vi "lvlauncher.vi"   [LabVIEW 2013]
uses:
  constants/arguments.ctl
  kernel32.dll
types:
  T1 = typedef "arguments.ctl" = cluster{"working directory":string, "flags":string[], "values":string[]}
  T2 = enum32{"invalid app kind", "Development System", "Run Time System", "Student Edition", "Embedded LabVIEW", "Evaluation", "Custom"}
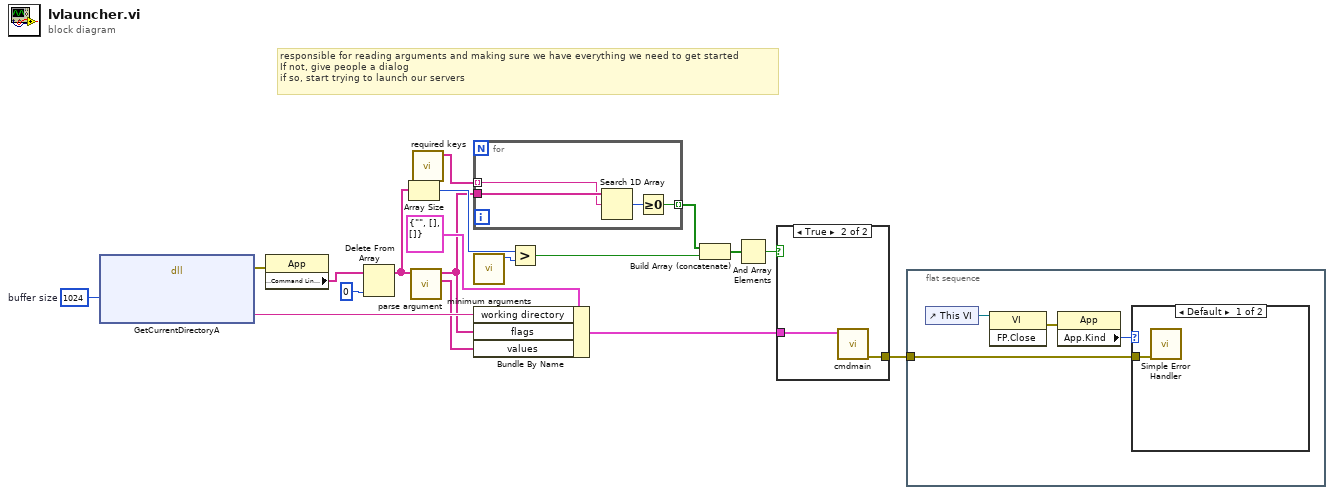
[diagram p0: block diagram]
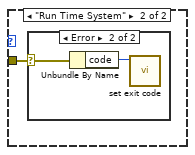
[diagram p2: hidden frame]
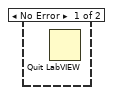
[diagram p3: hidden frame]
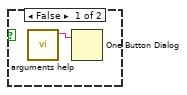
[diagram p4: hidden frame]
diagram:
  w17 = 1024  # buffer size
  # "responsible for reading arguments and making sure we have everything we need to get started\nIf not, give people a dialog\nif so, start trying to launch our servers"
  n1 = dll-call lib="kernel32.dll" fn="GetCurrentDirectoryA" ("Kernel32.dll - \nGetCurrentDirectoryA")("nBufferLength"=w17) -> (error out=w15:errorcluster, "lpBuffer"=w4:string)  [unwired: 5 in, 2 out]
  n2 = property class="App"(error in=w15) -> ("Application:Command Line Arguments"=w18:string[])  [unwired: 1 in, 2 out]
  n3 = Delete From Array(array=w18, index=0) -> (array with subset deleted=w11:string[])  [unwired: 1 in, 1 out]
  n4 = Array Size(array=w11) -> (size(s)=w12:i32)
  n5 = call "parse argument.vi"("Arguments"=w11) -> ("values"=w1:string[], "flags"=w2:string[])  [unwired: 9 in]
  n6 = call "required keys.vi"() -> ("required keys"=w10:string[])  [unwired: 11 in]
  n7 = for {
    tunnel: w2 -> [w22]
    tunnel: w10 -> [w21] mode=indexing
    tunnel: [w19] -> w9 mode=indexing
    n8 = Search 1D Array(1D array=w22, element=w21) -> (index of element=w20:i32)  [unwired: 1 in]
    n9 = Greater Or Equal To 0?(x=w20) -> (x >= 0?=w19:bool)
  }
  n10 = call "minimum arguments.vi"() -> ("minimum arguments"=w13:i32)  [unwired: 11 in]
  n11 = Bundle By Name(cluster=T1 {"working directory"="", "flags"=[], "values"=[]} ("command line arguments"), "working directory"=w4, "flags"=w2, "values"=w1) -> (w3:T1)
  n12 = Greater?(x=w12, y=w13) -> (0:w7:bool)
  n13 = Build Array (concatenate)(w9, w7) -> (w8:bool[])
  n14 = And Array Elements(Boolean array=w8) -> (logical AND=w6:bool)
  n15 = case shown="True" w6 {
    tunnel: [_ w25] -> w14
    tunnel: w3 -> [_ w24]
    frame False {
      n16 = call "arguments help.vi"() -> ("args help"=w23:string)  [unwired: 11 in]
      n17 = One Button Dialog(message=w23) -> ()  [unwired: 1 in, 1 out]
    }
    frame True {
      n18 = call "cmdmain.vi"("command line arguments"=w24) -> ("error out"=w25:errorcluster)  [unwired: 10 in]
    }
  }
  n19 = flat-sequence {
    tunnel: w14 -> [w26]
    frame #0 {
      n20 = control-ref of="This VI"() -> (w27:refnum<vi>)
      n21 = invoke class="VI" method="FP.Close"(reference=w27) -> (error out=w28:errorcluster)  [unwired: 2 in, 2 out]
      n22 = property class="App"(error in=w28) -> ("App.Kind"=w29:T2)  [unwired: 1 in, 2 out]
      n23 = case shown="Default" w29 {
        tunnel: w26 -> [w30 w31]
        frame Default {
          n24 = call <vilib>:"Simple Error Handler.vi"("error in (no error)"=w30) -> ()  [unwired: 4 in, 5 out]
        }
        frame "Run Time System" {
          n25 = case shown="Error" w31 {
            selector: w31 -> [_ w33]
            frame No Error {
              n26 = Quit LabVIEW() -> ()  [unwired: 1 in]
            }
            frame Error {
              n27 = Unbundle By Name(w33) -> ("code"=w32:i32)
              n28 = call "set exit code.vi"("exit code"=w32) -> ()  [unwired: 11 in]
            }
          }
        }
      }
    }
  }
